vi "Flush Queue of All But Priority Messages.vi"(8 "error in":errorcluster, 10 "priority messages":string[](array[string])=["Exit"], 11 "queue in":refnum<queue>) -> (0 "error out":errorcluster, 3 "queue out":refnum<queue>)   [LabVIEW 2024, in "DSA_CFG_ACQ.lvlib" / "SFPMessage Queue.lvlib"]
doc: "Clears the queue of all elements but those wired into the Priority Messages control."
uses:
  SFPMessage Queue.lvlib
  Message Cluster.ctl
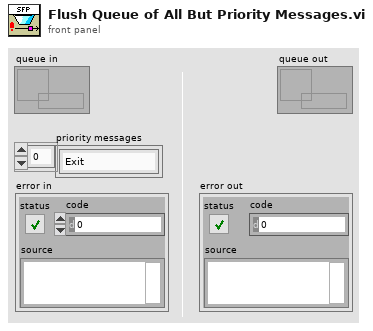
[diagram p1: front panel]
types:
  T1 = typedef "DSA_CFG_ACQ.lvlib/SFPMessage Queue.lvlib/Message Cluster.ctl" = cluster{"Message":string, "Message Data":variant}
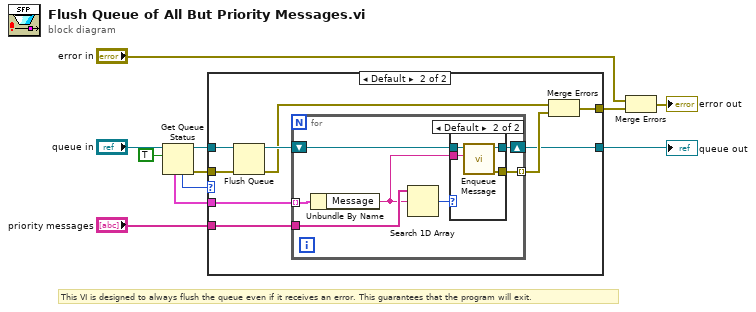
[diagram p0: block diagram]
diagram:
  # "This VI is designed to always flush the queue even if it receives an error. This guarantees that the program will exit."
  n1 = Get Queue Status(queue="queue in", return elements? (F)=TRUE) -> (queue out=w8:refnum<queue>, error out=w9:errorcluster, # elements in queue=w11:i32, elements=w7:T1[])  [unwired: 1 in, 4 out]
  n2 = case shown="Default" w11 {
    tunnel: w7 -> [_ w22]
    tunnel: w8 -> [w12 w21]
    tunnel: w9 -> [w13 w20]
    tunnel: [w13 w15] -> w3
    tunnel: "priority messages" -> [_ w18]
    tunnel: [w12 w14] -> w4
    frame 0 {
    }
    frame Default {
      n3 = Flush Queue(queue=w21, error in (no error)=w20) -> (queue out=w19:refnum<queue>, error out=w16:errorcluster)  [unwired: 1 out]
      n4 = for {
        tunnel: w22 -> [w29] mode=indexing
        tunnel: w18 -> [w27]
        tunnel: [w25] -> w17 mode=indexing
        shift-right: [w23] -> w14
        shift-left: w19 -> [w28]
        n5 = Unbundle By Name(w29) -> ("Message"=w26:string)
        n6 = Search 1D Array(1D array=w27, element=w26) -> (index of element=w24:i32)  [unwired: 1 in]
        n7 = case shown="Default" w24 {
          tunnel: w28 -> [w30 w34]
          tunnel: w26 -> [_ w33]
          tunnel: [_ w32] -> w25
          tunnel: [w30 w31] -> w23
          frame -1 {
          }
          frame Default {
            n8 = call "Enqueue Message.vi"("message"=w33, "message queue"=w34) -> ("error out"=w32:errorcluster, "dup message queue"=w31:refnum<queue>)  [unwired: 8 in]
          }
        }
      }
      n9 = Merge Errors(w16, w17) -> (w15:errorcluster)
    }
  }
  "queue out" <- w4
  n10 = Merge Errors("error in", w3) -> (→"error out":errorcluster)
